vi "VISA Command Test Panel.vi"() -> ()   [LabVIEW 2018]
panel:
  in  "Timeout(ms)":u32=3000
  out "Active":bool
  in  "stop":bool
  in  "Read":bool
  in  "Query":bool
  in  "Write":bool
  in  "Read byte count":u32=256
  in  "Command":string="*IDN?"
  out "Response":string
  in  "error in":errorcluster
  out "error out":errorcluster
  in  "VISA resource":refnum<visa-resource-name>="Scope1"
  # "Write + Read"
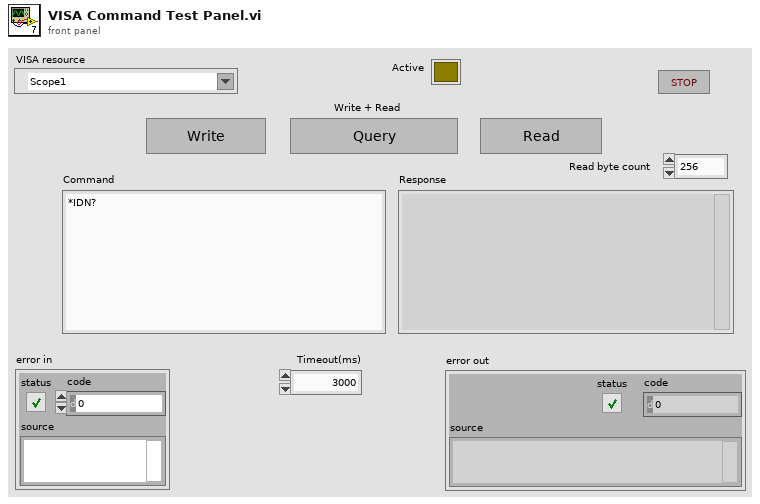
[diagram p1: front panel]
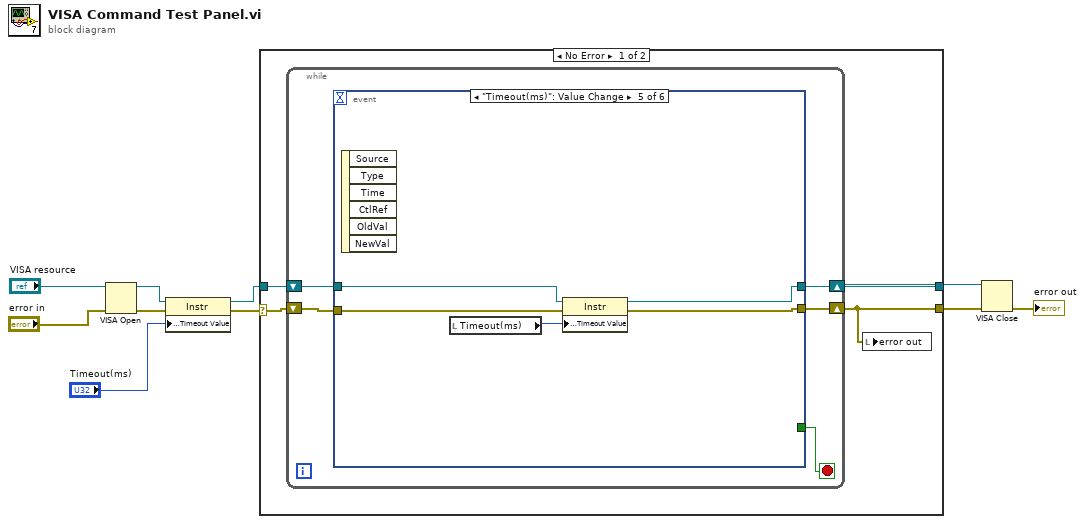
[diagram p0: block diagram]
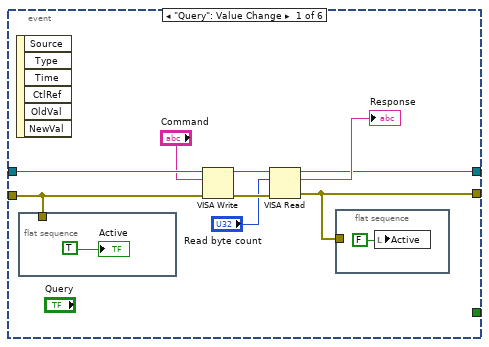
[diagram p2: hidden frame]
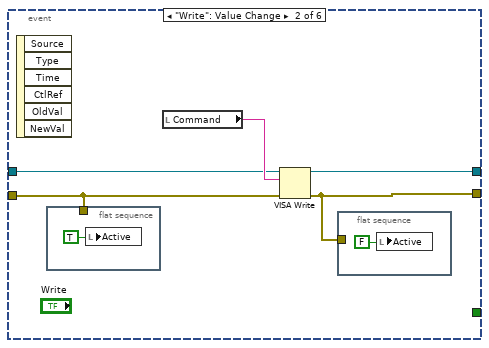
[diagram p3: hidden frame]
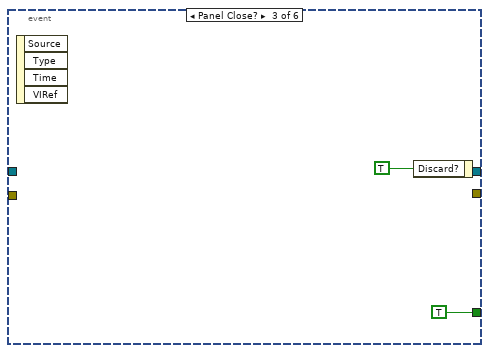
[diagram p4: hidden frame]
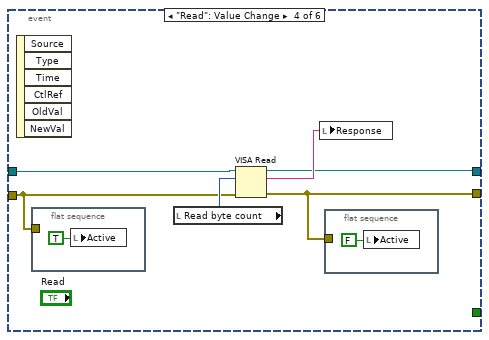
[diagram p5: hidden frame]
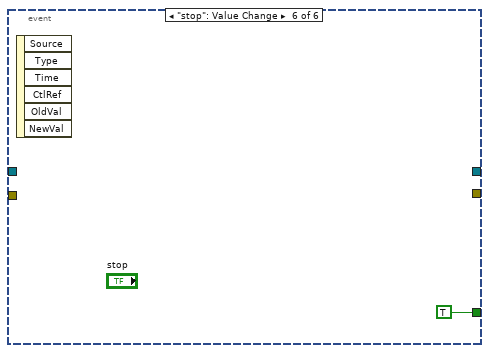
[diagram p6: hidden frame]
diagram:
  n1 = VISA Open(error in (no error)="error in", VISA resource name="VISA resource") -> (VISA resource name=w4:refnum<visa-resource-name>, error out=w2:errorcluster)  [unwired: 3 in]
  n2 = property class="Instr"(reference=w4, error in=w2, "General Settings:Timeout Value"="Timeout(ms)") -> (reference out=w1:refnum<visa-resource-name>, error out=w3:errorcluster)
  n3 = case shown="No Error" w3 {
    selector: w3 -> [w12 w55]
    tunnel: [w14 w54] -> w9
    tunnel: [w11 w55] -> w8
    tunnel: w1 -> [w13 w54]
    frame No Error {
      n4 = while {
        shift-right: [w19] -> w14
        shift-left: w13 -> [w17]
        shift-right: [w18] -> w11
        shift-left: w12 -> [w16]
        stop <- w15 stop-if-true
        n5 = event shown="[4] \"Timeout(ms)\": Value Change" {
          selector: _ -> [_ _ _ _ _ _]
          dyn-events: _ -> [_ _ _ _ _ _]
          timeout: _ -> [_ _ _ _ _ _]
          tunnel: [w27 w34 _ w42 w50 _] -> w19
          tunnel: [w20 w32 _ w41 w51 _] -> w18
          tunnel: w16 -> [w21 w31 _ w40 w48 _]
          tunnel: w17 -> [w24 w33 _ w45 w49 _]
          tunnel: [_ _ TRUE _ _ TRUE] -> w15
          event "Query": Value Change {
            n6 = event-data() -> ()  [unwired: 1 in, 6 out]
            n7 = flat-sequence {
              tunnel: w21 -> [_]
              frame #0 {
                "Active" <- TRUE
              }
            }
            n8 = VISA Write(VISA resource name=w24, write buffer="Command", error in (no error)=w21) -> (VISA resource name out=w26:refnum<visa-resource-name>, error out=w25:errorcluster)  [unwired: 1 out]
            n9 = VISA Read(VISA resource name=w26, byte count="Read byte count", error in (no error)=w25) -> (VISA resource name out=w27:refnum<visa-resource-name>, read buffer=→"Response":string, error out=w20:errorcluster)  [unwired: 1 out]
            n10 = flat-sequence {
              tunnel: w20 -> [_]
              frame #0 {
                n11 = local write "Active"(FALSE) -> ()
              }
            }
          }
          event "Write": Value Change {
            n12 = event-data() -> ()  [unwired: 1 in, 6 out]
            n13 = flat-sequence {
              tunnel: w31 -> [_]
              frame #0 {
                n14 = local write "Active"(TRUE) -> ()
              }
            }
            n15 = local read "Command"() -> (w35:string)
            n16 = VISA Write(VISA resource name=w33, write buffer=w35, error in (no error)=w31) -> (VISA resource name out=w34:refnum<visa-resource-name>, error out=w32:errorcluster)  [unwired: 1 out]
            n17 = flat-sequence {
              tunnel: w32 -> [_]
              frame #0 {
                n18 = local write "Active"(FALSE) -> ()
              }
            }
          }
          event Panel Close? {
            n19 = event-data() -> ()  [unwired: 1 in, 4 out]
            n20 = event-data("Discard?"=TRUE) -> ()  [unwired: 1 in, 1 out]
          }
          event "Read": Value Change {
            n21 = event-data() -> ()  [unwired: 1 in, 6 out]
            n22 = flat-sequence {
              tunnel: w40 -> [_]
              frame #0 {
                n23 = local write "Active"(TRUE) -> ()
              }
            }
            n24 = local read "Read byte count"() -> (w44:u32)
            n25 = VISA Read(VISA resource name=w45, byte count=w44, error in (no error)=w40) -> (VISA resource name out=w42:refnum<visa-resource-name>, read buffer=w43:string, error out=w41:errorcluster)  [unwired: 1 out]
            n26 = local write "Response"(w43) -> ()
            n27 = flat-sequence {
              tunnel: w41 -> [_]
              frame #0 {
                n28 = local write "Active"(FALSE) -> ()
              }
            }
          }
          event "Timeout(ms)": Value Change {
            n29 = event-data() -> ()  [unwired: 1 in, 6 out]
            n30 = local read "Timeout(ms)"() -> (w52:u32)
            n31 = property class="Instr"(reference=w49, error in=w48, "General Settings:Timeout Value"=w52) -> (reference out=w50:refnum<visa-resource-name>, error out=w51:errorcluster)
          }
          event "stop": Value Change {
            n32 = event-data() -> ()  [unwired: 1 in, 6 out]
          }
        }
      }
      n33 = local write "error out"(w11) -> ()
    }
    frame Error {
    }
  }
  n34 = VISA Close(VISA resource name=w9, error in (no error)=w8) -> (error out=→"error out":errorcluster)
